vi "verify related subimage parameters.vi"(8 "error in (no error)":errorcluster, 11 "Simulated_CCD_Camera in":refnum<class "Simulated Camera.lvclass">) -> (0 "error out":errorcluster, 3 "Simulated_CCD_Camera out":refnum<class "Simulated Camera.lvclass">)   [LabVIEW 2018, in "Simulated Camera.lvclass"]
doc: "Verify the related parameters of the camera\n\nThere are some parameters of the camera operation mode that depend on the value provided for another parameter. This function verifies if these parameters are in agreement."
uses:
  Simulated Camera.lvclass
  Simulated Camera.lvclass/Simulated Camera.ctl
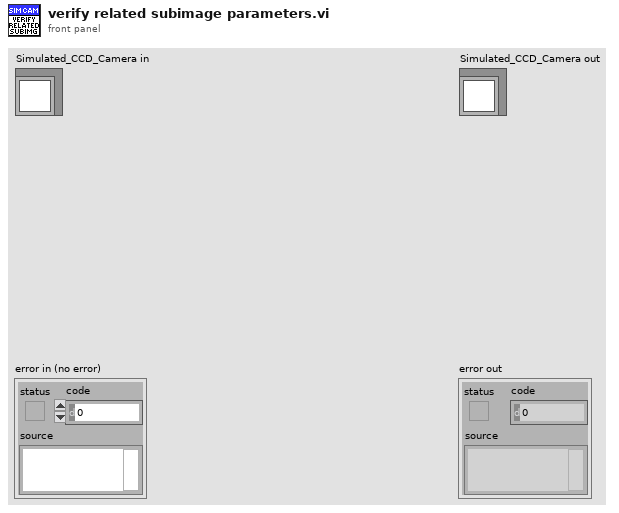
[diagram p1: front panel]
types:
  T1 = cluster{"PREAMP":u16, "READOUT_RATE":u16, "EM_GAIN":u16, "VERTICAL_SHIFT_SPEED":u16, "READ_MODE":u16, "FRAME_TRANSFER":bool, "VERTICAL_CLOCK_VOLTAGE":u16, "ACQUISITION_MODE":u16, "AD_CHANNEL":u16, "EM_MODE":u16, "SHUTTER_TTL":u16, "SHUTTER_OPENING_TIME":u16, "SHUTTER_CLOSING_TIME":u16, "SHUTTER_MODE":u16, "TRIGGER_MODE":u16, "VBIN":u16, "INITIAL_LINE":u16, "INITIAL_COLUMN":u16, "FINAL_LINE":u16, "FINAL_COLUMN":u16, "HBIN":u16}
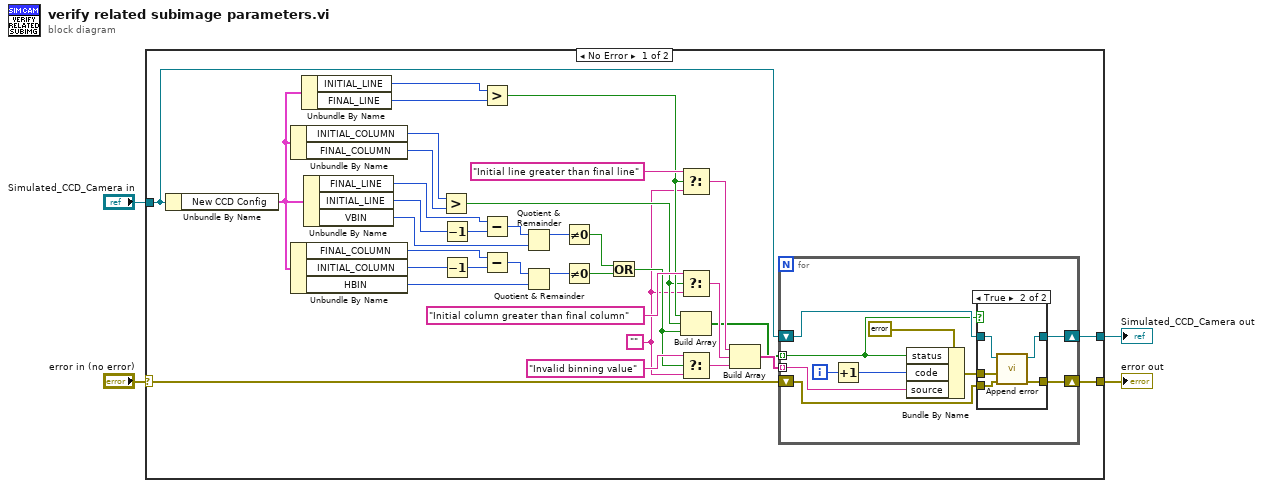
[diagram p0: block diagram]
diagram:
  n1 = case shown="No Error" "error in (no error)" {
    selector: "error in (no error)" -> [w7 w58]
    tunnel: [w6 w58] -> w3
    tunnel: [w8 w57] -> w1
    tunnel: "Simulated_CCD_Camera in" -> [w5 w57]
    frame No Error {
      w11 = ""
      n2 = Unbundle By Name(w5) -> ("New CCD Config"=w10:T1)
      n3 = Unbundle By Name(w10) -> ("INITIAL_COLUMN"=w36:u16, "FINAL_COLUMN"=w37:u16)
      n4 = Unbundle By Name(w10) -> ("FINAL_COLUMN"=w19:u16, "INITIAL_COLUMN"=w18:u16, "HBIN"=w17:u16)
      n5 = Unbundle By Name(w10) -> ("INITIAL_LINE"=w39:u16, "FINAL_LINE"=w38:u16)
      n6 = Unbundle By Name(w10) -> ("FINAL_LINE"=w35:u16, "INITIAL_LINE"=w29:u16, "VBIN"=w33:u16)
      n7 = Greater?(x=w36, y=w37) -> (0:w23:bool)
      n8 = Decrement(x=w29) -> (x-1=w28:u16)
      n9 = Decrement(x=w18) -> (x-1=w21:u16)
      n10 = Greater?(x=w39, y=w38) -> (0:w24:bool)
      n11 = Subtract(x=w35, y=w28) -> (x-y=w34:u16)
      n12 = Subtract(x=w19, y=w21) -> (x-y=w20:u16)
      n13 = Quotient & Remainder(x=w34, y=w33) -> (x-y*floor(x/y)=w12:u16)  [unwired: 1 out]
      n14 = Quotient & Remainder(x=w20, y=w17) -> (x-y*floor(x/y)=w13:u16)  [unwired: 1 out]
      n15 = Not Equal To 0?(x=w12) -> (x != 0?=w15:bool)
      n16 = Not Equal To 0?(x=w13) -> (x != 0?=w14:bool)
      n17 = Or(x=w15, y=w14) -> (x .or. y?=w16:bool)
      n18 = Select(t="Initial line greater than final line", s=w24, f=w11) -> (s? t:f=w27:string)
      n19 = Select(t="Initial column greater than final column", s=w23, f=w11) -> (s? t:f=w26:string)
      n20 = Build Array(w24, w23, w16) -> (w9:bool[])
      n21 = Select(t="Invalid binning value", s=w16, f=w11) -> (s? t:f=w25:string)
      n22 = Build Array(w27, w26, w25) -> (w22:string[])
      n23 = for {
        tunnel: w22 -> [w49] mode=indexing
        tunnel: w9 -> [w42] mode=indexing
        shift-right: [w48] -> w8
        shift-left: w5 -> [w47]
        shift-right: [w45] -> w6
        shift-left: w7 -> [w46]
        i -> [w44]
        n24 = Increment(x=w44) -> (x+1=w43:i32)
        n25 = Bundle By Name(cluster=errorcluster {"status"=FALSE, "code"=0, "source"=""} ("error constant"), "status"=w42, "code"=w43, "source"=w49) -> (w40:errorcluster)
        n26 = case shown="True" w42 {
          tunnel: [w51 w56] -> w48
          tunnel: w47 -> [w51 w55]
          tunnel: w46 -> [w50 w54]
          tunnel: [w50 w53] -> w45
          tunnel: w40 -> [_ w52]
          frame False {
          }
          frame True {
            n27 = call "Append error.vi"("error in (no error)"=w54, "error"=w52, "Simulated_CCD_Camera in"=w55) -> ("error out"=w53:errorcluster, "Simulated_CCD_Camera out"=w56:refnum<class "Simulated Camera.lvclass">)  [unwired: 7 in]
          }
        }
      }
    }
    frame Error {
    }
  }
  "error out" <- w3
  "Simulated_CCD_Camera out" <- w1
